vi "FRCts_ClientAPI_Interpret Header.vi"(8 "error in (no error)":errorcluster, 11 "Header":string="HTTP/1.1 301 Moved Permanently\r\nLocation: http://www.google.com/\r\nContent-Type: text/html; charset=UTF-8\r\nDate: Thu, 22 Mar 2012 21:41:48 GMT\r\nExpires: Sat, 21 Apr 2012 21:41:48 GMT\r\nCache-Control: public, max-age=2592000\r\nServer: gws\r\nContent-Length: 219\r\nX-XSS-Protection: 1; mode=block\r\nX-Frame-Options: SAMEORIGIN") -> (0 "error out":errorcluster, 1 "HTTP Response":string, 3 "HTTP Code":i32)   [LabVIEW 2014, in "FRCts_ClientAPI.lvlib"]
doc: "This VI interprets the header returned from HTTP actions."
uses:
  FRCts_ClientAPI.lvlib
  FRCts_ClientAPI_HTTP Header.ctl
panel:
  out "Header Values":T1[](array[typedef])
  out "HTTP Version":dbl
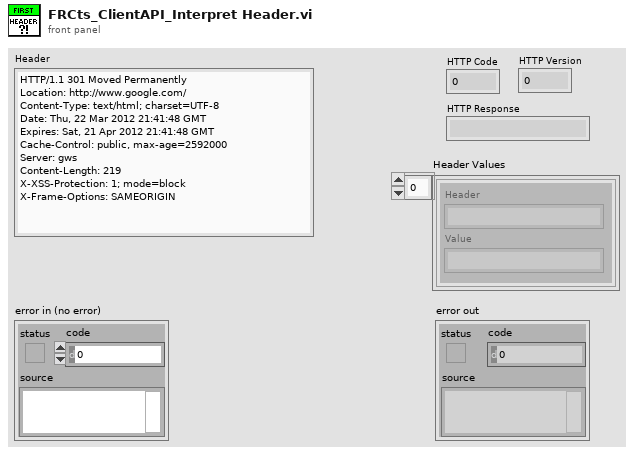
[diagram p1: front panel]
types:
  T1 = typedef "FRCts_ClientAPI.lvlib/FRCts_ClientAPI_HTTP Header.ctl" = cluster{"Header":string, "Value":string}
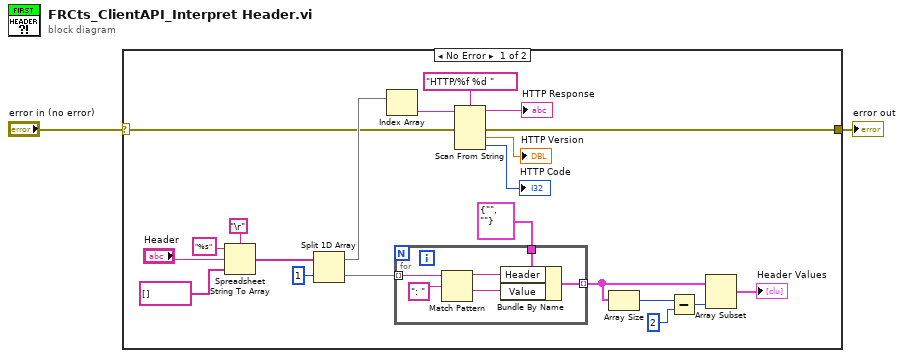
[diagram p0: block diagram]
diagram:
  n1 = case shown="No Error" "error in (no error)" {
    selector: "error in (no error)" -> [w11 w30]
    tunnel: [w10 w30] -> w1
    frame No Error {
      n2 = Spreadsheet String To Array(delimiter (Tab)="\r", format string="%s", spreadsheet string="Header", array type (2D Dbl)=string[] []) -> (array=w19:string[])
      n3 = Split 1D Array(array=w19, index=1) -> (first subarray=w17:string[], second subarray=w12:string[])
      n4 = Index Array(array=w17) -> (element=w16:string)  [unwired: 1 in]
      n5 = for {
        tunnel: w12 -> [w29] mode=indexing
        tunnel: T1 {"Header"="", "Value"=""} ("HTTP Header") -> [w27]
        tunnel: [w24] -> w8 mode=indexing
        n6 = Match Pattern(string=w29, regular expression=": ") -> (before substring=w26:string, after substring=w25:string)  [unwired: 1 in, 2 out]
        n7 = Bundle By Name(cluster=w27, "Header"=w26, "Value"=w25) -> (w24:T1)
      }
      n8 = Scan From String(format string="HTTP/%f %d ", input string=w16, error in=w11) -> (remaining string=→"HTTP Response":string, error out=w10:errorcluster, output 1=→"HTTP Version":dbl, output 2=→"HTTP Code":i32)  [unwired: 3 in, 1 out]
      n9 = Array Size(array=w8) -> (size(s)=w7:i32)
      n10 = Subtract(x=w7, y=2) -> (x-y=w9:i32)
      n11 = Array Subset(array=w8, length=w9) -> (→"Header Values":T1[])  [unwired: 1 in]
    }
    frame Error {
    }
  }
  "error out" <- w1
